vi "mxwScript_API_Option_DropRelation.vi"(7 "direction":T1, 8 "error in (no error)":errorcluster, 9 "addWireSpace":bool=TRUE, 10 "distance":i32 min=0, 11 "options in":T2[](array[typedef])) -> (0 "error out":errorcluster, 3 "options out":T2[](array[typedef]))   [LabVIEW 2017]
doc: "Sets the default relationship between the template and block diagram reference points. This is used to calculate the drop position of templates."
uses:
  codeGenAPISupport.llb/cgAPI_mxwScript_OptionData.ctl
  codeGenAPISupport.llb/cgAPI_mxwScript_DrpTmplt_SimpleDirection.ctl
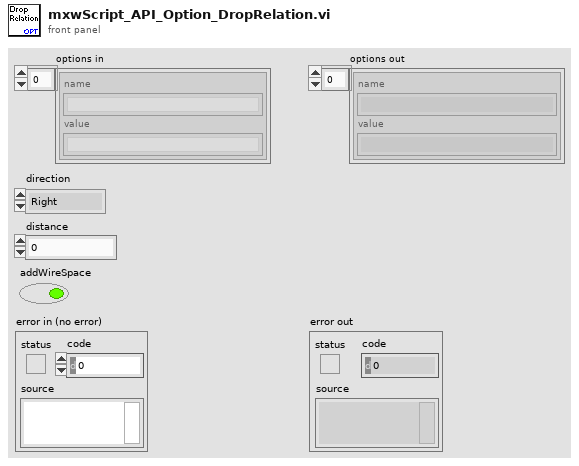
[diagram p1: front panel]
types:
  T1 = typedef "cgAPI_mxwScript_DrpTmplt_SimpleDirection.ctl" = enum16{"Right", "Left", "Below", "Above"}
  T2 = typedef "cgAPI_mxwScript_OptionData.ctl" = cluster{"name":string, "value":string}
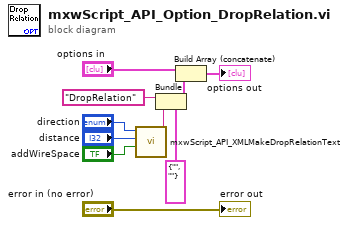
[diagram p0: block diagram]
diagram:
  n1 = call "mxwScript_API_XMLMakeDropRelationText.vi"("addWireSpace"="addWireSpace", "distance"="distance", "direction"="direction") -> ("XML out"=w2:string)  [unwired: 8 out]
  n2 = Bundle(cluster=T2 {"name"="", "value"=""} ("optionData"), "name"="DropRelation", "value"=w2) -> (w8:T2)
  n3 = Build Array (concatenate)("options in", w8) -> (→"options out":T2[])
  "error out" <- "error in (no error)"
